vi "Example Match Pattern Demo.vi"() -> ()   [LabVIEW 2014]
uses:
  vi.lib/Q-WaveSystems/QwaveSys Raspberry Pi for LabVIEW Home-Education/QwaveSys Raspberry Pi Library.lvlib
panel:
  out "score":dbl
  out "2D Picture":picture
  out "Template":picture
  out "Output":picture
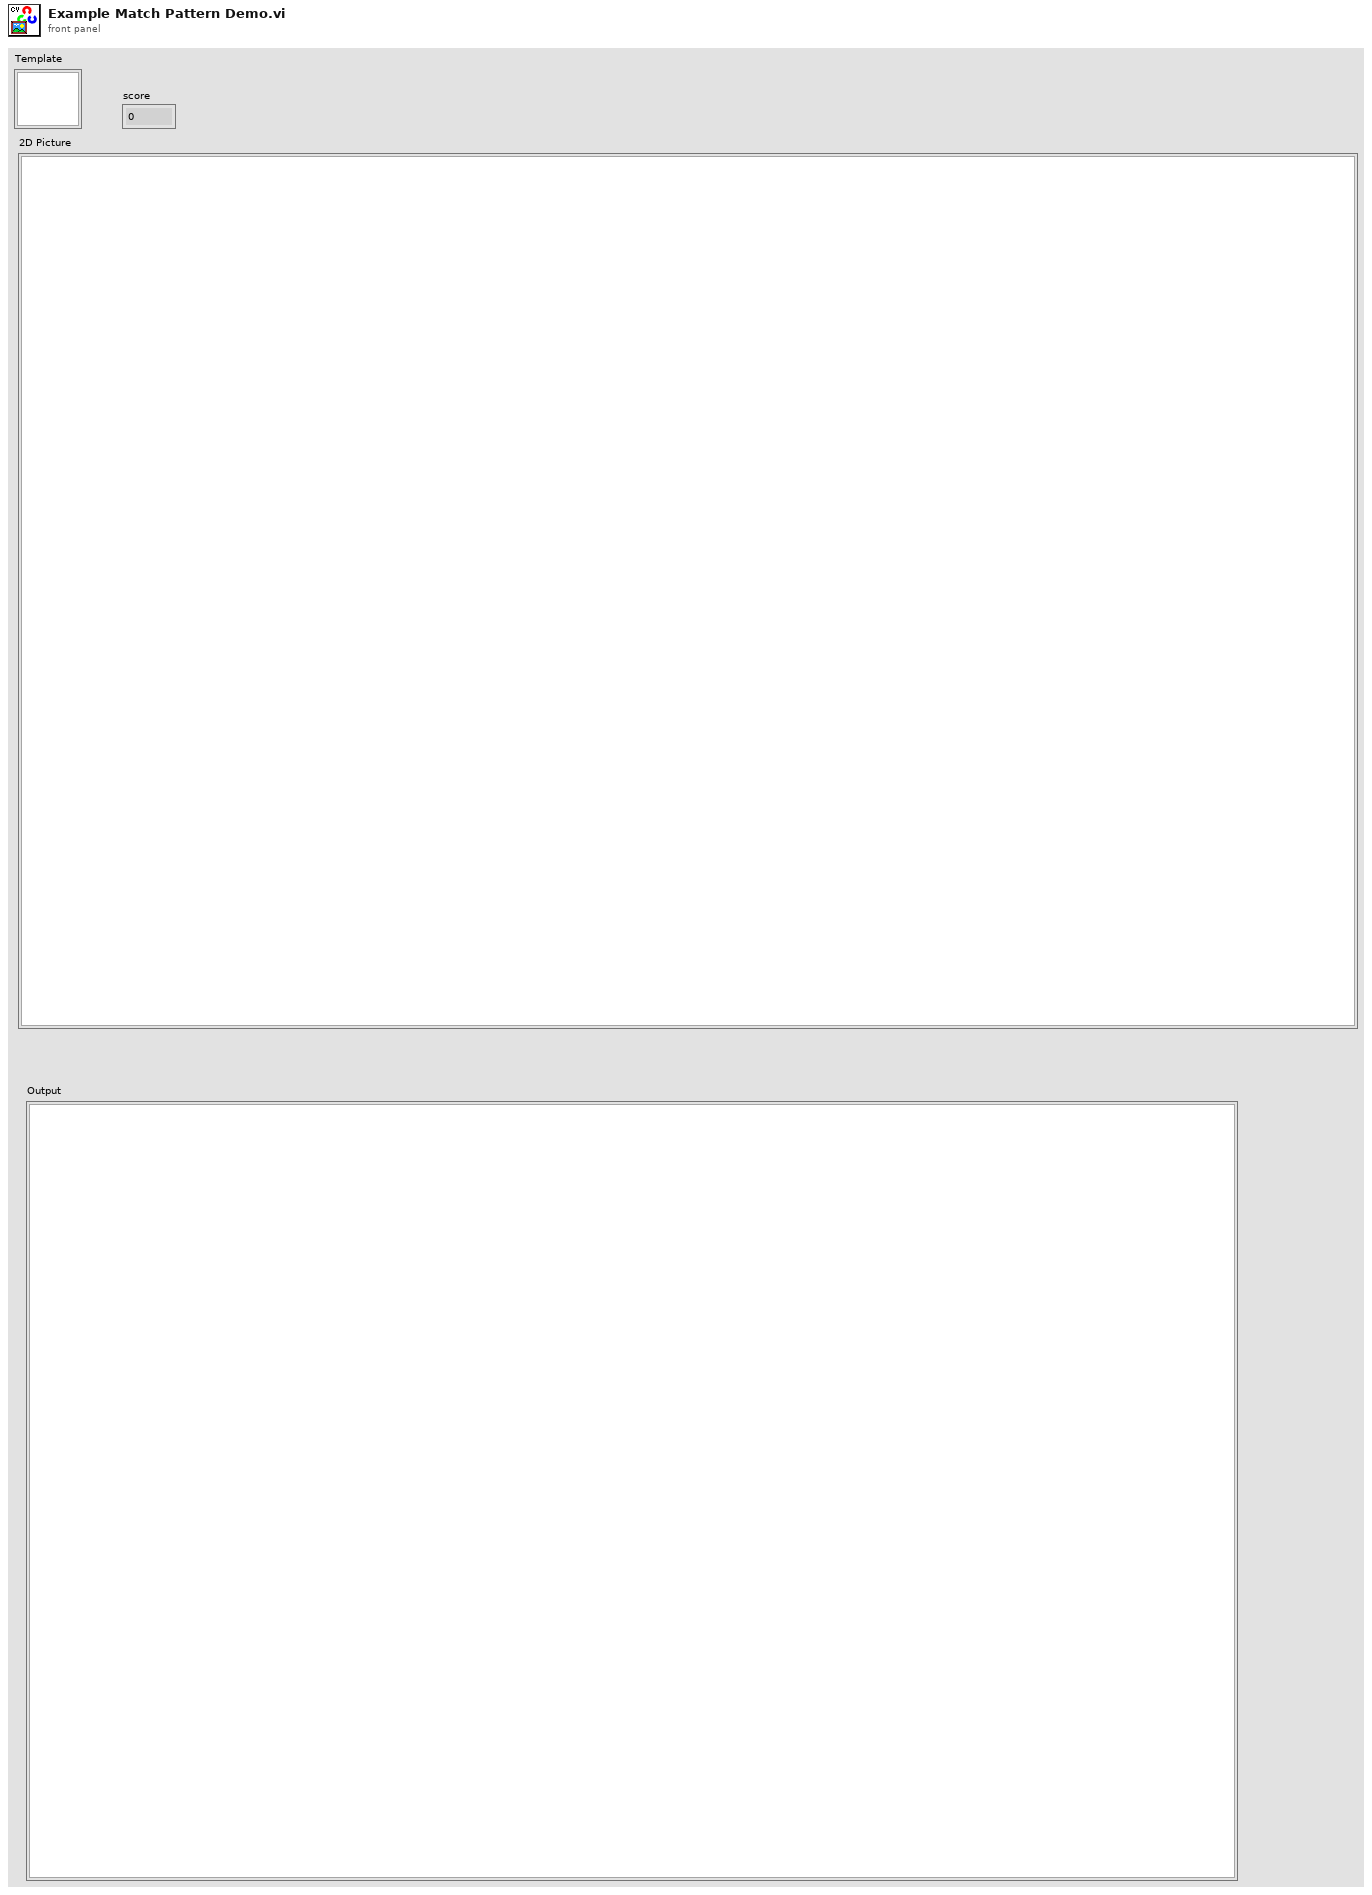
[diagram p1: front panel]
types:
  T1 = typedef "imagedata.ctl" = cluster{"image type":i32, "image depth":i32, "image":u8[], "mask":u8[], "colors":u32[], "Rectangle":cluster{"left":i16, "top":i16, "right":i16, "bottom":i16}}
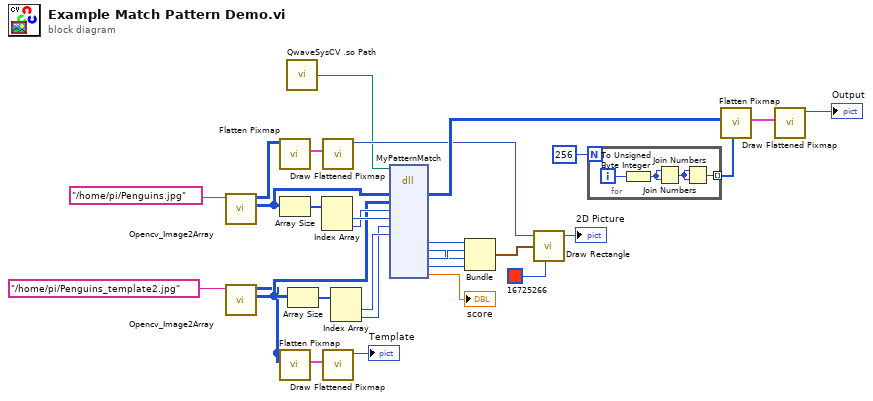
[diagram p0: block diagram]
diagram:
  n1 = call "Opencv_Image2Array.vi"("filename"="/home/pi/Penguins.jpg") -> ("Image Pixels Gray"=w24:u8[][], "Image Pixels 24 bits"=w12:u32[][])  [unwired: 8 in, 1 out]
  n2 = call "Opencv_Image2Array.vi"("filename"="/home/pi/Penguins_template2.jpg") -> ("Image Pixels Gray"=w23:u8[][], "Image Pixels 24 bits"=w2:u32[][])  [unwired: 8 in, 1 out]
  n3 = call <vilib>:"Flatten Pixmap.vi"("24-bit pixmap"=w12) -> ("image data"=w13:T1)  [unwired: 10 in]
  n4 = Array Size(array=w24) -> (size(s)=w30:i32[])
  n5 = call <vilib>:"Flatten Pixmap.vi"("8-bit pixmap"=w2, "24-bit pixmap"=w2) -> ("image data"=w18:T1)  [unwired: 9 in]
  n6 = call "QwaveSysCV .so Path.vi"() -> ("QwaveSys .so Path"=w1:path)  [unwired: 5 in]
  n7 = Array Size(array=w23) -> (size(s)=w27:i32[])
  n8 = Index Array(array=w30) -> (element #1=w29:i32, element #2=w28:i32)  [unwired: 2 in]
  n9 = call <vilib>:"Draw Flattened Pixmap.vi"("image data"=w13) -> ("new picture"=w5:picture)  [unwired: 8 in]
  n10 = call <vilib>:"Draw Flattened Pixmap.vi"("image data"=w18) -> ("new picture"=→"Template":picture)  [unwired: 8 in]
  n11 = Index Array(array=w27) -> (element #1=w26:i32, element #2=w25:i32)  [unwired: 2 in]
  n12 = dll-call lib="libqwavesys.so" fn="MyPatternMatch"(path in=w1, "src"=w24, "templ"=w23, "src_cols"=w28, "src_rows"=w29, "templ_cols"=w25, "templ_rows"=w26) -> ("src"=w15:u8[][], "xL"=w10:i32, "xR"=w8:i32, "yT"=w9:i32, "yB"=w7:i32, "score"=→"score":dbl)  [unwired: 13 in, 2 out]
  n13 = Bundle("xL"=w10, "yT"=w9, "xR"=w8, "yB"=w7) -> (w11:cluster{"xL":i32, "yT":i32, "xR":i32, "yB":i32})  [unwired: 1 in]
  n14 = call <vilib>:"Draw Rectangle.vi"("picture"=w5, "rect"=w11, "color(black)"=u32 16725266) -> ("new picture"=→"2D Picture":picture)  [unwired: 6 in]
  n15 = for {
    N: 256 -> [_]
    tunnel: [w34] -> w14 mode=indexing
    i -> [w32]
    n16 = To Unsigned Byte Integer(number=w32) -> (unsigned 8bit integer=w31:u8)
    n17 = Join Numbers(hi=w31, lo=w31) -> ((hi.lo)=w33:u16)
    n18 = Join Numbers(hi=w33, lo=w33) -> ((hi.lo)=w34:u32)
  }
  n19 = call <vilib>:"Flatten Pixmap.vi"("colors"=w14, "8-bit pixmap"=w15) -> ("image data"=w20:T1)  [unwired: 9 in]
  n20 = call <vilib>:"Draw Flattened Pixmap.vi"("image data"=w20) -> ("new picture"=→"Output":picture)  [unwired: 8 in]
